vi "Keithley 6517 Trace Buffer Store and Read.vi"() -> ()   [LabVIEW 2016]
doc: "Stores the specified number of readings in the buffer from the specified soure and reads them along with buffer statistics.\n\n<B>Note:</B>\nThis VI is compatible with both 6514 and 6517."
uses:
  <instrlib>/Keithley 6517/Keithley 6517.lvlib
panel:
  in  "Timeout (10000 ms)":u32=10000
  out "Peak-to-Peak":dbl
  out "Mean":dbl
  out "Standard Deviation":dbl
  out "Maximum":dbl
  out "Minimum":dbl
  out "Measurements":T1(array[cluster]) {"Measurement" format="%.6e"}
  in  "Buffer Time Stamp Format (0: Absolute)":i32(ring) items=["Absolute", "Delta"]
  in  "Buffer Size (10)":i32=10
  in  "Buffer Source (0: Raw Input Readings)":u16(ring) items=["Raw Input Readings", "CALC1 Readings", "CALC2 Readings"]
  in  "VISA resource name":refnum<visa-resource-name>
  # "(c) 2016-2017 National Instruments.  ALL RIGHTS RESERVED."
  # "Note: This Example is compatible with both 6517 and 6514 models."
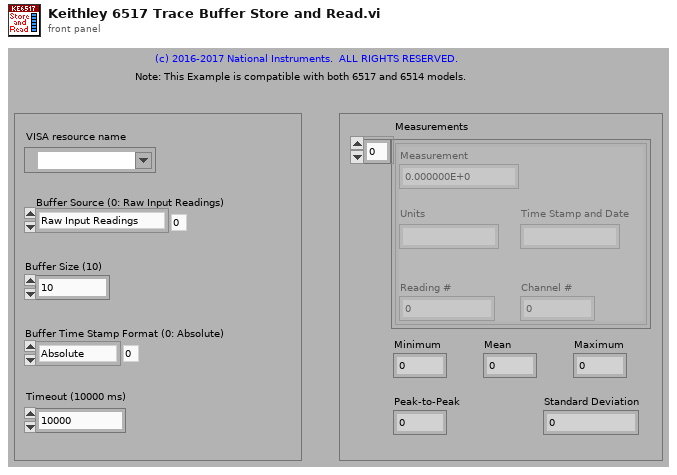
[diagram p1: front panel]
types:
  T1 = cluster{"Measurement":dbl, "Units":string, "Time Stamp and Date":string, "Reading #":dbl, "Channel #":dbl}[]
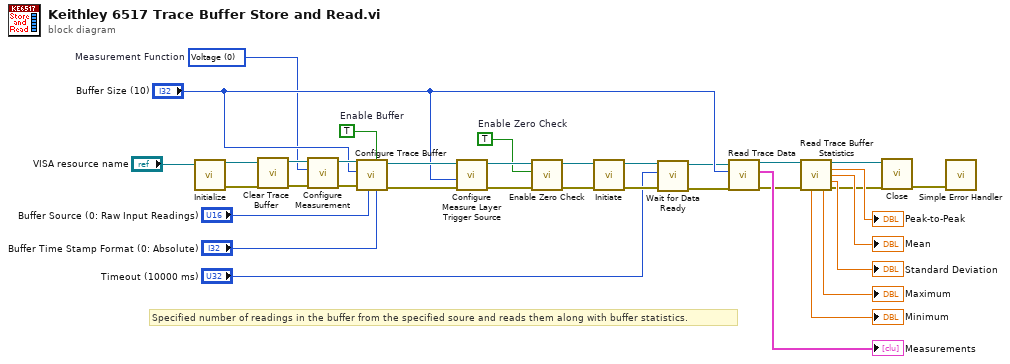
[diagram p0: block diagram]
diagram:
  w11 = 0 items=["Voltage", "Current", "Resistance", "Charge"]  # Measurement Function
  w17 = TRUE  # Enable Zero Check
  w31 = TRUE  # Enable Buffer
  # "Specified number of readings in the buffer from the specified soure and reads them along with buffer statistics."
  n1 = call <instrlib>:"Initialize.vi"("VISA resource name"="VISA resource name") -> ("error out"=w9:errorcluster, "VISA resource name out"=w10:refnum<visa-resource-name>)  [unwired: 9 in]
  n2 = call <instrlib>:"Clear Trace Buffer.vi"("error in (no error)"=w9, "VISA resource name"=w10) -> ("error out"=w24:errorcluster, "VISA resource name out"=w25:refnum<visa-resource-name>)  [unwired: 8 in]
  n3 = call <instrlib>:"Configure Measurement.vi"("error in (no error)"=w24, "Measurement Function (0: Voltage)"=w11, "VISA resource name"=w25) -> ("error out"=w22:errorcluster, "VISA resource name out"=w23:refnum<visa-resource-name>)  [unwired: 7 in]
  n4 = call <instrlib>:"Configure Trace Buffer.vi"("Buffer Time Stamp Format (0: Absolute)"="Buffer Time Stamp Format (0: Absolute)", "Enable Buffer (0: Disable)"=w31, "Buffer Source (0: Raw Input Readings)"="Buffer Source (0: Raw Input Readings)", "error in (no error)"=w22, "Buffer Size (100)"="Buffer Size (10)", "VISA resource name"=w23) -> ("error out"=w15:errorcluster, "VISA resource name out"=w16:refnum<visa-resource-name>)  [unwired: 4 in]
  n5 = call <instrlib>:"Configure Measure Layer Trigger Source.vi"("error in (no error)"=w15, "Measure Count (1)"="Buffer Size (10)", "VISA resource name"=w16) -> ("error out"=w20:errorcluster, "VISA resource name out"=w21:refnum<visa-resource-name>)  [unwired: 7 in]
  n6 = call <instrlib>:"Enable Zero Check.vi"("error in (no error)"=w20, "Enable Zero Check (T: Enable)"=w17, "VISA resource name"=w21) -> ("error out"=w18:errorcluster, "VISA resource name out"=w19:refnum<visa-resource-name>)  [unwired: 7 in]
  n7 = call <instrlib>:"Initiate.vi"("error in (no error)"=w18, "VISA resource name"=w19) -> ("error out"=w7:errorcluster, "VISA resource name out"=w8:refnum<visa-resource-name>)  [unwired: 8 in]
  n8 = call <instrlib>:"Wait for Data Ready.vi"("error in (no error)"=w7, "Timeout (10000 ms)"="Timeout (10000 ms)", "VISA resource name"=w8) -> ("error out"=w5:errorcluster, "VISA resource name out"=w6:refnum<visa-resource-name>)  [unwired: 7 in]
  n9 = call <instrlib>:"Read Trace Data.vi"("error in (no error)"=w5, "Count Value (1)"="Buffer Size (10)", "VISA resource name"=w6) -> ("error out"=w13:errorcluster, "Measurements"=→"Measurements":T1, "VISA resource name out"=w14:refnum<visa-resource-name>)  [unwired: 6 in]
  n10 = call <instrlib>:"Read Trace Buffer Statistics.vi"("VISA resource name"=w14, "error in (no error)"=w13) -> ("Maximum"=→"Maximum":dbl, "VISA resource name out"=w3:refnum<visa-resource-name>, "Peak-to-Peak"=→"Peak-to-Peak":dbl, "Mean"=→"Mean":dbl, "Standard Deviation"=→"Standard Deviation":dbl, "Minimum"=→"Minimum":dbl, "error out"=w2:errorcluster)  [unwired: 7 in]
  n11 = call <instrlib>:"Close.vi"("error in (no error)"=w2, "VISA resource name"=w3) -> ("error out"=w1:errorcluster)  [unwired: 9 in]
  n12 = call <vilib>:"Simple Error Handler.vi"("error in (no error)"=w1) -> ()  [unwired: 4 in, 5 out]
